vi "Subspaces Angle.vi"   [LabVIEW 2020, in "NI_AAL_LinAlg.lvlib"]
doc: "Computes the angle between column spaces of two matrices."
uses:
  <vilib>/Analysis/NI_AAL_LinAlg.lvlib
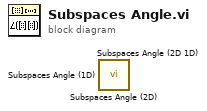
[diagram p0: block diagram]
diagram:
  n1 = call <vilib>:"Subspaces Angle (2D).vi"() -> ()  [unwired: 10 in, 2 out]
  n2 = call <vilib>:"Subspaces Angle (2D 1D).vi"() -> ()  [unwired: 10 in, 2 out]
  n3 = call <vilib>:"Subspaces Angle (1D).vi"() -> ()  [unwired: 10 in, 2 out]
